vi "PlotDataGen.vi"(11 "AllData":dbl[][](array[numeric])) -> (2 "Y Data":dbl[][](array[numeric]), 3 "XData":dbl[](array[numeric]))   [LabVIEW 2010]
panel:
  out "Graphe XY":cluster{"AllData":dbl[], dbl[]}[](graph)
  out "XY Graph":T1(array[cluster])
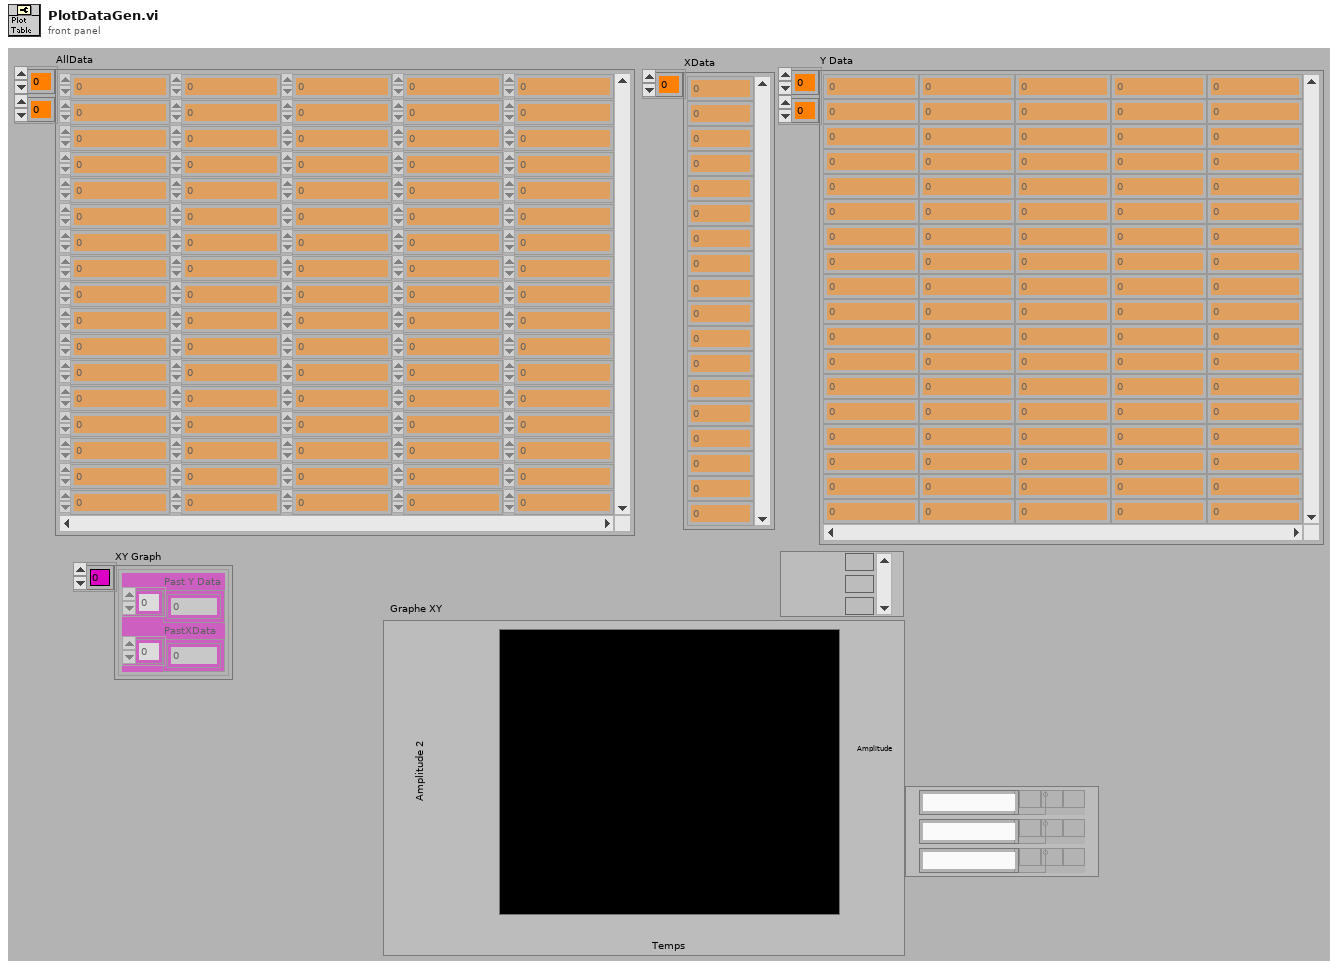
[diagram p1: front panel]
types:
  T1 = cluster{"Past Y Data":dbl[], "PastXData":dbl[]}[]
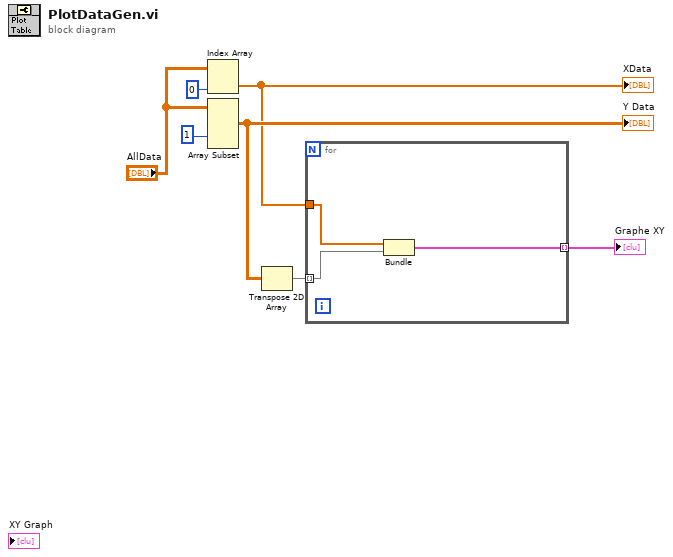
[diagram p0: block diagram]
diagram:
  n1 = Index Array(array="AllData", index (col)=0 ("indice désactivé (col)")) -> (element=w3:dbl[])  [unwired: 1 in]
  "XData" <- w3
  n2 = Array Subset(array="AllData", index (col)=1 ("indice")) -> (w4:dbl[][])  [unwired: 3 in]
  "Y Data" <- w4
  n3 = Transpose 2D Array(2D array=w4) -> (transposed array=w1:dbl[][])
  n4 = for {
    tunnel: w1 -> [w9] mode=indexing
    tunnel: w3 -> [w10]
    tunnel: [w8] -> w2 mode=indexing
    n5 = Bundle("AllData"=w10, w9) -> (w8:cluster{"AllData":dbl[], dbl[]})  [unwired: 1 in]
  }
  "Graphe XY" <- w2
